vi "Structure Handler.vi"() -> ()   [LabVIEW 2010] (continued)
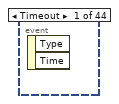
[diagram p4: hidden frame]
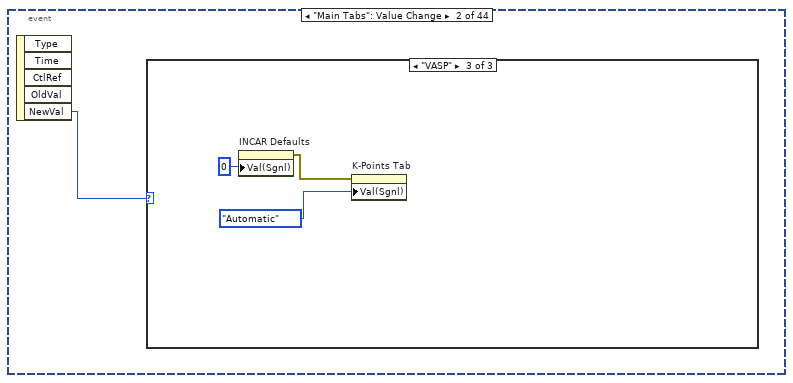
[diagram p5: hidden frame]
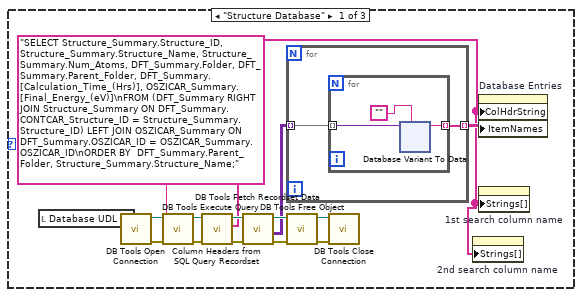
[diagram p6: hidden frame]
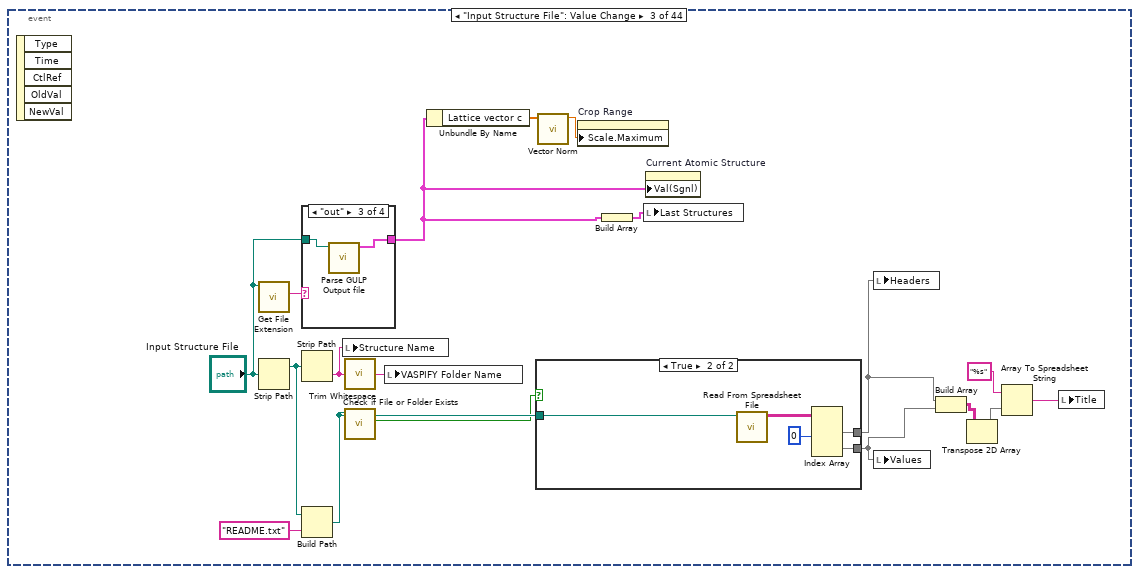
[diagram p8: hidden frame]
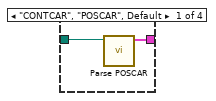
[diagram p10: hidden frame]
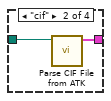
[diagram p11: hidden frame]
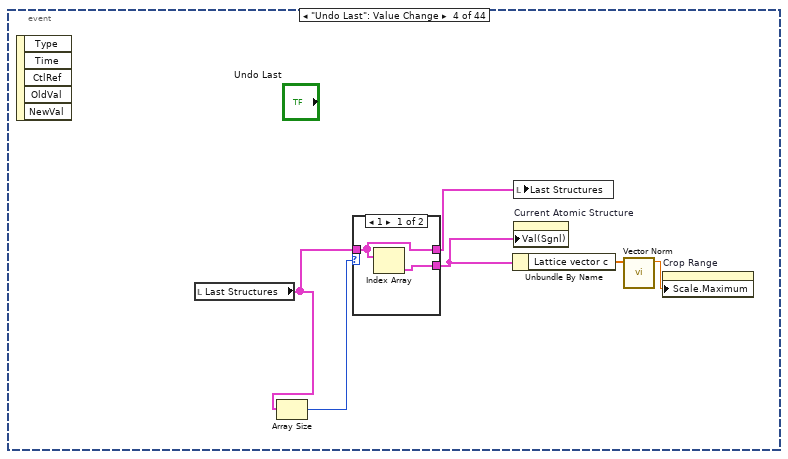
[diagram p13: hidden frame]
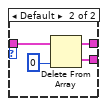
[diagram p14: hidden frame]
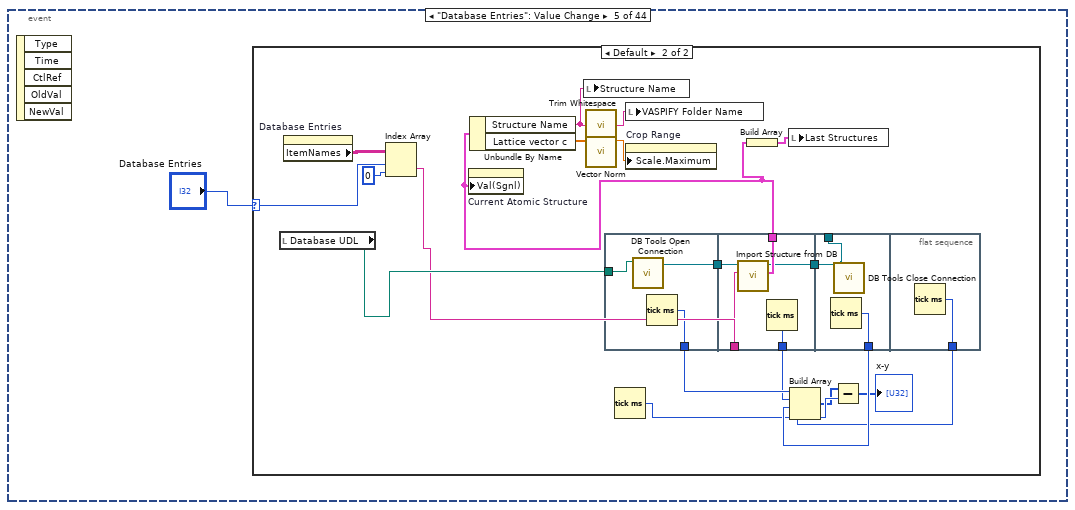
[diagram p15: hidden frame]
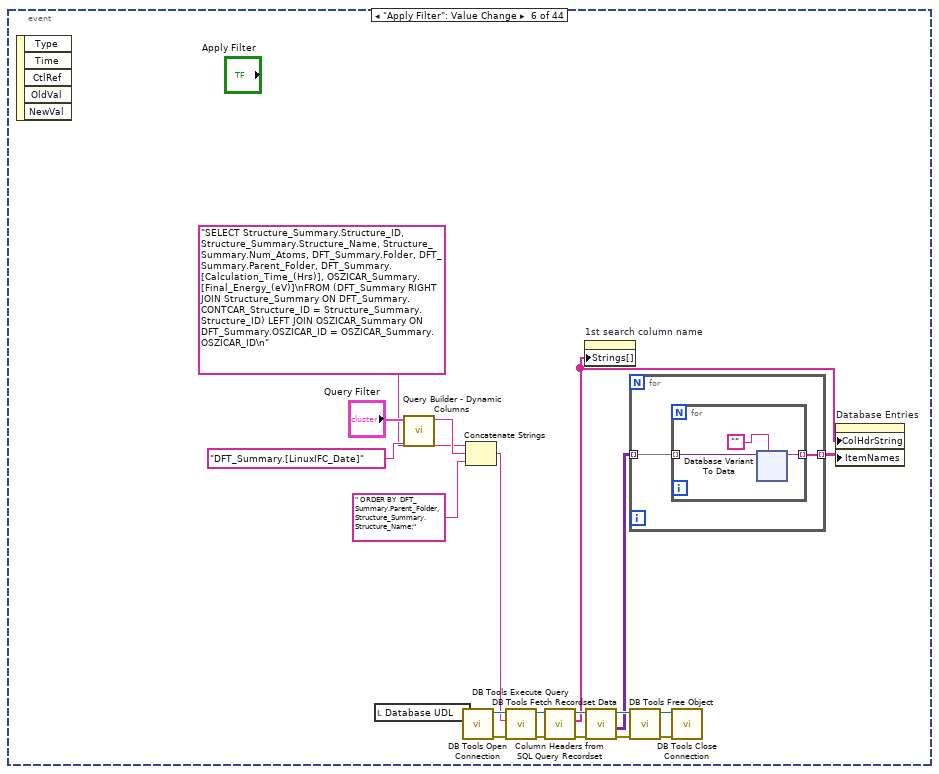
[diagram p17: hidden frame]
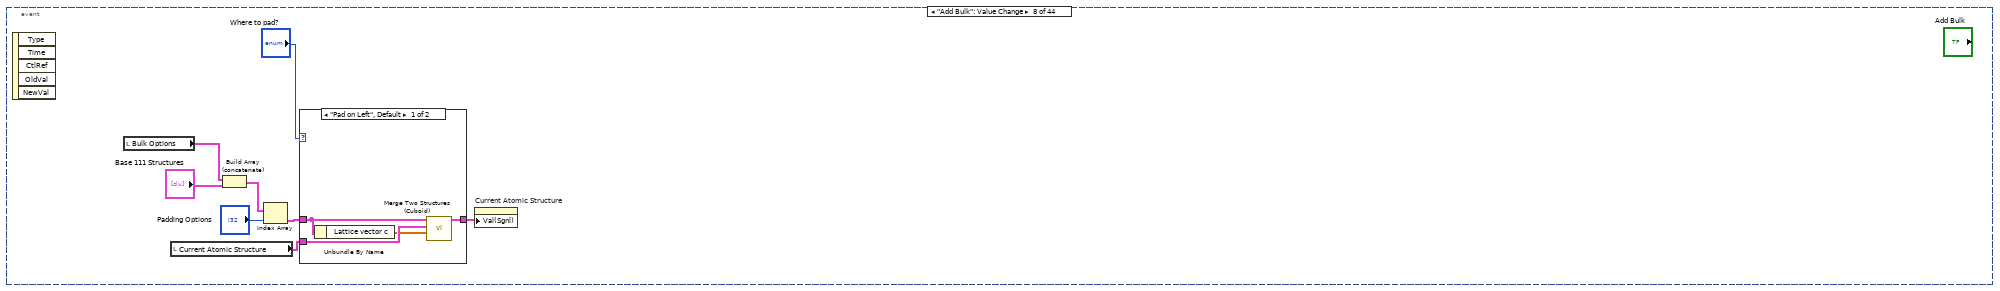
[diagram p19: hidden frame]
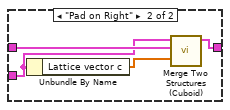
[diagram p20: hidden frame]
                  }
                  frame True {
                    n569 = local read "Atom List"() -> (w1005:i32[])
                    n570 = Search 1D Array(1D array=w1005, element=w1004) -> (index of element=w1003:i32)  [unwired: 1 in]
                    n571 = case shown="Default" w1003 {
                      tunnel: [w1007 w1010] -> w1006
                      tunnel: w1005 -> [w1007 w1009]
                      tunnel: w1004 -> [_ w1008]
                      frame Default {
                      }
                      frame -1 {
                        n572 = Build Array (concatenate)(w1009, w1008) -> (w1010:i32[])
                      }
                    }
                  }
                }
                n573 = property on="Atom List" class="MCListbox (strict)"("Val(Sgnl)"=w986) -> ()  [unwired: 2 in, 2 out]
              }
            }
          }
        }
      }
      event "Make Vacancy": Value Change {
        n574 = event-data() -> ()  [unwired: 1 in, 5 out]
        n575 = local read "Current Atomic Structure"() -> (w1031:T3)
        n576 = Unbundle By Name(w1031) -> ("Atoms Array"=w1032:T20, "# of atoms"=w1028:i32)
        n577 = local read "Atom List"() -> (w1030:i32[])
        n578 = for {
          tunnel: w1032 -> [w1057] mode=indexing
          tunnel: w1030 -> [w1059]
          tunnel: [w1053] -> w1025 mode=indexing
          shift-right: [w1051] -> _
          shift-left: 0 -> [w1052]
          w1058 = dbl[][] []
          n579 = Unbundle By Name(w1057) -> ("Atom Name"=w1056:string, "Positions (Direct)"=w1061:dbl[][], "Positions (Cartesian)"=w1060:dbl[][])
          n580 = for {
            tunnel: w1061 -> [w1069] mode=indexing
            tunnel: w1060 -> [w1066] mode=indexing
            tunnel: w1059 -> [w1071]
            shift-right: [w1065] -> w1054
            shift-left: w1058 -> [w1064]
            shift-right: [w1068] -> w1055
            shift-left: w1058 -> [w1067]
            shift-right: [w1063] -> w1051
            shift-left: w1052 -> [w1062]
            n581 = Search 1D Array(1D array=w1071, element=w1062) -> (index of element=w1070:i32)  [unwired: 1 in]
            n582 = Increment(x=w1062) -> (x+1=w1063:i32)
            n583 = case shown="Default" w1070 {
              tunnel: w1069 -> [_ w1079]
              tunnel: [w1073 w1078] -> w1068
              tunnel: w1067 -> [w1073 w1077]
              tunnel: w1066 -> [_ w1076]
              tunnel: [w1072 w1075] -> w1065
              tunnel: w1064 -> [w1072 w1074]
              frame Default {
              }
              frame -1 {
                n584 = Build Array (concatenate)(w1077, w1079) -> (w1078:dbl[][])
                n585 = Build Array (concatenate)(w1074, w1076) -> (w1075:dbl[][])
              }
            }
          }
          n586 = Bundle(cluster=w1057, "Atom Name"=w1056, "Positions (Direct)"=w1055, "Positions (Cartesian)"=w1054) -> (w1053:T23)
        }
        n587 = Array Size(array=w1030) -> (size(s)=w1029:i32)
        n588 = Subtract(x=w1028, y=w1029) -> (x-y=w1027:i32)
        n589 = Bundle By Name(cluster=w1031, "Atoms Array"=w1025, "# of atoms"=w1027) -> (w1026:T3)
        n590 = local read "Headers"() -> (w1020:string[])
        n591 = local read "Values"() -> (w1021:string[])
        n592 = property on="Current Atomic Structure" class="Clust (strict)"("Val(Sgnl)"=w1026) -> ()  [unwired: 2 in, 2 out]
        n593 = for {
          tunnel: string[] ["Defect Name", "Location"] -> [w1035] mode=indexing
          shift-right: [w1036] -> w1022
          shift-left: w1020 -> [w1037]
          shift-right: [w1033] -> w1023
          shift-left: w1021 -> [w1038]
          tunnel: string[] ["Vacancy", ""] -> [w1034] mode=indexing
          n594 = Search 1D Array(1D array=w1037, element=w1035) -> (index of element=w1039:i32)  [unwired: 1 in]
          n595 = case shown="-1" w1039 {
            selector: w1039 -> [w1043 _]
            tunnel: w1038 -> [w1044 w1047]
            tunnel: [w1042 w1045] -> w1033
            tunnel: w1037 -> [w1041 w1050]
            tunnel: [w1041 w1048] -> w1036
            tunnel: w1035 -> [_ w1049]
            tunnel: w1034 -> [w1040 w1046]
            frame Default {
              n596 = Replace Array Subset(array=w1044, new element=w1040, index=w1043) -> (w1042:string[])
            }
            frame -1 {
              n597 = Build Array (concatenate)(w1047, w1046) -> (w1045:string[])
              n598 = Build Array (concatenate)(w1050, w1049) -> (w1048:string[])
            }
          }
        }
        n599 = local write "Values"(w1023) -> ()
        n600 = local write "Headers"(w1022) -> ()
      }
      event "Replace Atom": Value Change {
        w1088 = dbl[][] []
        n601 = event-data() -> ()  [unwired: 1 in, 5 out]
        n602 = local read "Current Atomic Structure"() -> (w1099:T3)
        n603 = local read "Atom List"() -> (w1098:i32[])
        n604 = Unbundle By Name(w1099) -> ("Atoms Array"=w1100:T20)
        n605 = for {
          tunnel: w1100 -> [w1150] mode=indexing
          tunnel: w1098 -> [w1151]
          tunnel: [w1146] -> w1095 mode=indexing
          shift-right: [w1144] -> _
          shift-left: 0 -> [w1145]
          shift-right: [w1142] -> w1090
          shift-left: w1088 -> [w1140]
          shift-right: [w1141] -> w1089
          shift-left: w1088 -> [w1139]
          w1143 = dbl[][] []
          n606 = Unbundle By Name(w1150) -> ("Atom Name"=w1149:string, "Positions (Direct)"=w1153:dbl[][], "Positions (Cartesian)"=w1152:dbl[][])
          n607 = for {
            tunnel: w1153 -> [w1165] mode=indexing
            tunnel: w1152 -> [w1162] mode=indexing
            tunnel: w1151 -> [w1167]
            shift-right: [w1161] -> w1147
            shift-left: w1143 -> [w1160]
            shift-right: [w1164] -> w1148
            shift-left: w1143 -> [w1163]
            shift-right: [w1159] -> w1144
            shift-left: w1145 -> [w1158]
            shift-right: [w1157] -> w1142
            shift-left: w1140 -> [w1156]
            shift-right: [w1155] -> w1141
            shift-left: w1139 -> [w1154]
            n608 = Search 1D Array(1D array=w1167, element=w1158) -> (index of element=w1166:i32)  [unwired: 1 in]
            n609 = case shown="-1" w1166 {
              tunnel: w1165 -> [w1173 w1183]
              tunnel: [w1175 w1182] -> w1164
              tunnel: w1163 -> [w1175 w1181]
              tunnel: w1162 -> [w1170 w1180]
              tunnel: [w1174 w1179] -> w1161
              tunnel: w1160 -> [w1174 w1178]
              tunnel: [w1172 w1176] -> w1157
              tunnel: w1156 -> [w1171 w1176]
              tunnel: [w1169 w1177] -> w1155
              tunnel: w1154 -> [w1168 w1177]
              frame Default {
                n610 = Build Array (concatenate)(w1171, w1173) -> (w1172:dbl[][])
                n611 = Build Array (concatenate)(w1168, w1170) -> (w1169:dbl[][])
              }
              frame -1 {
                n612 = Build Array (concatenate)(w1181, w1183) -> (w1182:dbl[][])
                n613 = Build Array (concatenate)(w1178, w1180) -> (w1179:dbl[][])
              }
            }
            n614 = Increment(x=w1158) -> (x+1=w1159:i32)
          }
          n615 = Bundle(cluster=w1150, "Atom Name"=w1149, "Positions (Direct)"=w1148, "Positions (Cartesian)"=w1147) -> (w1146:T23)
        }
        n616 = for {
          tunnel: w1095 -> [w1128] mode=indexing
          tunnel: w1090 -> [w1127]
          tunnel: w1089 -> [w1126]
          tunnel: [w1125] -> w1094 mode=indexing
          tunnel: "Replacement Atom" -> [w1124]
          tunnel: [w1123] -> w1087 mode=indexing
          n617 = Unbundle By Name(w1128) -> ("Atom Name"=w1129:string)
          n618 = Equal?(x=w1124, y=w1129) -> (x = y?=w1123:bool)
          n619 = case shown="True" w1123 {
            tunnel: w1128 -> [w1130 w1134]
            tunnel: w1127 -> [_ w1137]
            tunnel: w1126 -> [_ w1135]
            tunnel: [w1130 w1131] -> w1125
            frame False {
            }
            frame True {
              n620 = Unbundle By Name(w1134) -> ("Positions (Direct)"=w1138:dbl[][], "Positions (Cartesian)"=w1136:dbl[][])
              n621 = Build Array (concatenate)(w1138, w1137) -> (w1132:dbl[][])
              n622 = Build Array (concatenate)(w1136, w1135) -> (w1133:dbl[][])
              n623 = Bundle By Name(cluster=w1134, "Positions (Direct)"=w1132, "Positions (Cartesian)"=w1133) -> (w1131:T23)
            }
          }
        }
        n624 = Bundle("Replacement Atom"="Replacement Atom", w1090, w1089) -> (w1091:T29)  [unwired: 1 in]
        n625 = Or Array Elements(Boolean array=w1087) -> (logical OR=w1086:bool)
        n626 = case shown="False" w1086 {
          tunnel: w1094 -> [w1121 w1122]
          tunnel: [w1120 w1122] -> w1093
          tunnel: w1091 -> [w1119 _]
          frame False {
            n627 = Build Array (concatenate)(w1121, w1119) -> (w1120:T30)
          }
          frame True {
          }
        }
        n628 = Bundle By Name(cluster=w1099, "Atoms Array"=w1093) -> (w1097:T3)
        n629 = property on="Current Atomic Structure" class="Clust (strict)"("Val(Sgnl)"=w1097) -> ()  [unwired: 2 in, 2 out]
        n630 = local read "Headers"() -> (w1082:string[])
        n631 = local read "Values"() -> (w1083:string[])
        n632 = for {
          tunnel: string[] ["Defect Name", "Location"] -> [w1103] mode=indexing
          shift-right: [w1104] -> w1084
          shift-left: w1082 -> [w1105]
          shift-right: [w1101] -> w1085
          shift-left: w1083 -> [w1106]
          tunnel: string[] ["Substitutional", ""] -> [w1102] mode=indexing
          n633 = Search 1D Array(1D array=w1105, element=w1103) -> (index of element=w1107:i32)  [unwired: 1 in]
          n634 = case shown="-1" w1107 {
            selector: w1107 -> [w1111 _]
            tunnel: w1106 -> [w1112 w1115]
            tunnel: [w1110 w1113] -> w1101
            tunnel: w1105 -> [w1109 w1118]
            tunnel: [w1109 w1116] -> w1104
            tunnel: w1103 -> [_ w1117]
            tunnel: w1102 -> [w1108 w1114]
            frame Default {
              n635 = Replace Array Subset(array=w1112, new element=w1108, index=w1111) -> (w1110:string[])
            }
            frame -1 {
              n636 = Build Array (concatenate)(w1115, w1114) -> (w1113:string[])
              n637 = Build Array (concatenate)(w1118, w1117) -> (w1116:string[])
            }
          }
        }
        n638 = local write "Values"(w1085) -> ()
        n639 = local write "Headers"(w1084) -> ()
      }
      event "Add Interstitial": Value Change {
        w1202 = dbl[] [0.0, 0.0, 0.0]
        n640 = event-data() -> ()  [unwired: 1 in, 5 out]
        n641 = local read "Current Atomic Structure"() -> (w1194:T3)
        n642 = local read "Headers"() -> (w1189:string[])
        n643 = local read "Values"() -> (w1188:string[])
        n644 = Unbundle By Name(w1194) -> ("Atoms Array"=w1203:T20, "# of atoms"=w1192:i32)
        n645 = for {
          tunnel: string[] ["Defect Name", "Location"] -> [w1207] mode=indexing
          shift-right: [w1208] -> w1187
          shift-left: w1189 -> [w1209]
          shift-right: [w1205] -> w1186
          shift-left: w1188 -> [w1210]
          tunnel: string[] ["Interstitial", ""] -> [w1206] mode=indexing
          n646 = Search 1D Array(1D array=w1209, element=w1207) -> (index of element=w1211:i32)  [unwired: 1 in]
          n647 = case shown="-1" w1211 {
            selector: w1211 -> [w1215 _]
            tunnel: w1210 -> [w1216 w1219]
            tunnel: [w1214 w1217] -> w1205
            tunnel: w1209 -> [w1213 w1222]
            tunnel: [w1213 w1220] -> w1208
            tunnel: w1207 -> [_ w1221]
            tunnel: w1206 -> [w1212 w1218]
            frame Default {
              n648 = Replace Array Subset(array=w1216, new element=w1212, index=w1215) -> (w1214:string[])
            }
            frame -1 {
              n649 = Build Array (concatenate)(w1219, w1218) -> (w1217:string[])
              n650 = Build Array (concatenate)(w1222, w1221) -> (w1220:string[])
            }
          }
        }
        n651 = local read "Atom List"() -> (w1190:i32[])
        n652 = for {
          tunnel: w1203 -> [w1229] mode=indexing
          tunnel: w1190 -> [w1230]
          shift-right: [w1223] -> _
          shift-left: 0 -> [w1228]
          shift-right: [w1227] -> w1200
          shift-left: w1202 -> [w1225]
          shift-right: [w1226] -> w1199
          shift-left: w1202 -> [w1224]
          tunnel: [w1223] -> _ mode=indexing
          n653 = Unbundle By Name(w1229) -> ("Positions (Direct)"=w1232:dbl[][], "Positions (Cartesian)"=w1231:dbl[][])  [unwired: 1 out]
          n654 = for {
            tunnel: w1232 -> [w1240] mode=indexing
            tunnel: w1231 -> [w1239] mode=indexing
            tunnel: w1230 -> [w1242]
            shift-right: [w1233] -> w1223
            shift-left: w1228 -> [w1238]
            shift-right: [w1237] -> w1227
            shift-left: w1225 -> [w1236]
            shift-right: [w1235] -> w1226
            shift-left: w1224 -> [w1234]
            n655 = Search 1D Array(1D array=w1242, element=w1238) -> (index of element=w1241:i32)  [unwired: 1 in]
            n656 = case shown="Default" w1241 {
              tunnel: w1240 -> [w1247 _]
              tunnel: w1239 -> [w1244 _]
              tunnel: [w1246 w1249] -> w1237
              tunnel: w1236 -> [w1248 w1249]
              tunnel: [w1243 w1250] -> w1235
              tunnel: w1234 -> [w1245 w1250]
              frame Default {
                n657 = Add(x=w1248, y=w1247) -> (x+y=w1246:dbl[])
                n658 = Add(x=w1245, y=w1244) -> (x+y=w1243:dbl[])
              }
              frame -1 {
              }
            }
            n659 = Increment(x=w1238) -> (x+1=w1233:i32)
          }
        }
        n660 = Array Size(array=w1190) -> (size(s)=w1198:i32)
        n661 = Increment(x=w1192) -> (x+1=w1191:i32)
        n662 = local write "Headers"(w1187) -> ()
        n663 = local write "Values"(w1186) -> ()
        n664 = local read "Replacement Atom"() -> (w1204:string)
        n665 = Divide(x=w1200, y=w1198) -> (x/y=w1197:dbl[])
        n666 = Divide(x=w1199, y=w1198) -> (x/y=w1196:dbl[])
        n667 = for {
          tunnel: w1203 -> [w1256] mode=indexing
          tunnel: w1197 -> [w1255]
          tunnel: w1196 -> [w1254]
          tunnel: [w1253] -> w1195 mode=indexing
          tunnel: w1204 -> [w1252]
          n668 = Unbundle By Name(w1256) -> ("Atom Name"=w1257:string)
          n669 = Equal?(x=w1252, y=w1257) -> (x = y?=w1251:bool)
          n670 = case shown="True" w1251 {
            tunnel: w1256 -> [w1258 w1262]
            tunnel: w1255 -> [_ w1265]
            tunnel: w1254 -> [_ w1263]
            tunnel: [w1258 w1259] -> w1253
            frame False {
            }
            frame True {
              n671 = Unbundle By Name(w1262) -> ("Positions (Direct)"=w1266:dbl[][], "Positions (Cartesian)"=w1264:dbl[][])
              n672 = Build Array (concatenate)(w1266, w1265) -> (w1260:dbl[][])
              n673 = Build Array (concatenate)(w1264, w1263) -> (w1261:dbl[][])
              n674 = Bundle By Name(cluster=w1262, "Positions (Direct)"=w1260, "Positions (Cartesian)"=w1261) -> (w1259:T23)
            }
          }
        }
        n675 = Bundle By Name(cluster=w1194, "Atoms Array"=w1195, "# of atoms"=w1191) -> (w1193:T3)
        n676 = property on="Current Atomic Structure" class="Clust (strict)"("Val(Sgnl)"=w1193) -> ()  [unwired: 2 in, 2 out]
      }
      event "Make defect pair": Value Change {
        n677 = event-data() -> ()  [unwired: 1 in, 5 out]
        n678 = local read "Current Atomic Structure"() -> (w1269:T3)
        n679 = call "Make Defect Pair.vi"("Maximum Distnce"="Maximum Distnce", "Minimum Distance"="Minimum Distance", "Defect 2"="Defect 2", "Defect 1"="Defect 1", "Defect 1 Atom Index"="Defect 1 Atom Index", "Input Structure"=w1269) -> ("Defectuous Structure"=w1270:T3)  [unwired: 2 in, 3 out]
        n680 = property on="Current Atomic Structure" class="Clust (strict)"("Val(Sgnl)"=w1270) -> ()  [unwired: 2 in, 2 out]
      }
      event "Max Bond Length", "Axis": Value Change {
        n681 = event-data() -> ()  [unwired: 1 in, 5 out]
        n682 = local read "Current Atomic Structure"() -> (w1278:T3)
        n683 = call "Find all Bonds in Structure.vi"("Max Bond Length"="Max Bond Length", "Structure"=w1278) -> ("Bonds"=w1277:T31)  [unwired: 9 in]
        n684 = for {
          tunnel: w1277 -> [w1285] mode=indexing
          tunnel: "Axis" -> [w1283]
          tunnel: [w1280] -> w1275 mode=indexing
          n685 = Unbundle By Name(w1285) -> ("Bond Center Position"=w1284:dbl[], "Bond Length (A)"=w1281:dbl)
          n686 = Index Array(array=w1284, index=w1283) -> (element=w1282:dbl)
          n687 = Bundle("Numeric"=w1282, "Bond Length (A)"=w1281) -> (w1280:cluster{"Numeric":dbl, "Bond Length (A)":dbl})  [unwired: 1 in]
        }
        n688 = Sort 1D Array(array=w1275) -> (sorted array=→"System XY Graph":cluster{"Numeric":dbl, "Bond Length (A)":dbl}[])
      }
      event "Map to [0,1)": Value Change {
        n689 = event-data() -> ()  [unwired: 1 in, 5 out]
        n690 = local read "Current Atomic Structure"() -> (w1287:T3)
        n691 = call "Map Structure to [0,1).vi"("Structure"=w1287) -> ("Structure mapped to [0,1)"=w1286:T32)  [unwired: 10 in]
        n692 = property on="Current Atomic Structure" class="Clust (strict)"("Val(Sgnl)"=w1286) -> ()  [unwired: 2 in, 2 out]
      }
      event "Remove Close Atoms": Value Change {
        n693 = event-data() -> ()  [unwired: 1 in, 5 out]
        n694 = local read "Current Atomic Structure"() -> (w1291:T3)
        n695 = call "Remove Close Atoms.vi"("Minimally Allowable Distance (A)"="Minimally Allowable Distance (A)", "Structure"=w1291) -> ("# of Atoms Removed"=→"# of Atoms Removed":i32, "Structure with atoms removed"=w1290:T3)  [unwired: 8 in]
        n696 = property on="Current Atomic Structure" class="Clust (strict)"("Val(Sgnl)"=w1290) -> ()  [unwired: 2 in, 2 out]
      }
      event "Load in VESTA": Value Change {
        n697 = event-data() -> ()  [unwired: 1 in, 5 out]
        n698 = local read "Current Atomic Structure"() -> (w1292:T3)
        n699 = call "Load Structure in VESTA.vi"("Atomic Structure"=w1292) -> ()  [unwired: 11 in]
      }
    }
  }
  n700 = call <vilib>:"Create Object.vi"("Name"="Base") -> ("error out"=w1:errorcluster, "Scene:New Object"=w2:refnum<vi>)  [unwired: 1 in, 8 out]
  n701 = local write "Base Object"(w2) -> ()
  n702 = disable-structure shown="Disabled" {
    disable-tunnel: w1 -> [w1294 _]
    frame Disabled {
      n703 = property on="Current Atomic Structure" class="Clust (strict)"(error in=w1294, "Val(Sgnl)"=T3 {"Structure Name"="(60.0) twist [1,1,1] [1,1,1+0.0tilt] (0.00,0.00,0.00)T GB", "Lattice vector a"=[4.678066827442777, 0.0, 0.0], "Lattice vector b"=[0.0, 8.10264942633344, 0.0], "Lattice vector c"=[0.0, 0.0, 23.0], "Atoms Array"=[{"Atom Name"="Cd", "Positions (Direct)"=[[0.0, 5.4807901278164903e-17, -0.000893984567927683], [0.0, 0.0, 0.4991060154320723], [0.0, 0.3333333333333333, 0.3321413539094297], [0.0, 0.6666666666666666, 0.16607067695471486], [0.4999999999999999, 0.16666666666666666, 0.16607067695471486], [0.5, 0.5, -0.000893984567927683], [0.5, 0.5, 0.4991060154320723], [0.4999999999999999, 0.8333333333333331, 0.3321413539094297], [0.9999999999999998, 0.3333333333333333, 0.3321413539094297], [0.9999999999999998, 0.6666666666666667, 0.16607067695471486], [0.0, 0.33333333333333326, 0.6660706769547148], [0.0, 0.6666666666666666, 0.8321413539094297], [0.5, 0.16666666666666674, 0.8321413539094297], [0.5, 0.8333333333333333, 0.6660706769547148]], "Positions (Cartesian)"=[[0.0, 4.440892098500626e-16, -0.02056164506233671], [0.0, 0.0, 11.479438354937663], [0.0, 2.700883142111146, 7.639251139916884], [0.0, 5.401766284222292, 3.819625569958442], [2.339033413721388, 1.350441571055573, 3.819625569958442], [2.3390334137213884, 4.05132471316672, -0.02056164506233671], [2.3390334137213884, 4.05132471316672, 11.479438354937663], [2.339033413721388, 6.752207855277865, 7.639251139916884], [4.678066827442776, 2.700883142111146, 7.639251139916884], [4.678066827442776, 5.401766284222293, 3.819625569958442], [0.0, 2.7008831421111457, 15.319625569958442], [0.0, 5.401766284222292, 19.139251139916883], [2.3390334137213884, 1.3504415710555737, 19.139251139916883], [2.3390334137213884, 6.752207855277866, 15.319625569958442]]}, {"Atom Name"="Te", "Positions (Direct)"=[[0.0, 0.0, 0.12455300771603617], [0.0, 0.33333333333333337, 0.45669436162546595], [0.0, 0.6666666666666666, 0.29062368467075106], [0.4999999999999999, 0.16666666666666663, 0.29062368467075106], [0.4999999999999999, 0.4999999999999999, 0.12455300771603621], [0.4999999999999999, 0.8333333333333331, 0.45669436162546595], [0.9999999999999998, 5.4807901278164903e-17, 0.12455300771603621], [0.9999999999999998, 0.3333333333333333, 0.45669436162546595], [0.9999999999999998, 0.6666666666666669, 0.29062368467075106], [0.0, 1.1331166295920983e-17, 0.6245530077160362], [0.0, 0.3333333333333333, 0.7906236846707511], [0.0, 0.6666666666666666, 0.9566943616254658], [0.0, 0.9999999999999998, 0.6245530077160362], [0.4999999999999999, 0.1666666666666668, 0.9566943616254658], [0.4999999999999999, 0.8333333333333334, 0.7906236846707511], [0.5000000000000001, 0.5, 0.6245530077160362]], "Positions (Cartesian)"=[[0.0, 0.0, 2.864719177468832], [0.0, 2.7008831421111466, 10.503970317385717], [0.0, 5.401766284222292, 6.684344747427274], [2.339033413721388, 1.3504415710555728, 6.684344747427275], [2.339033413721388, 4.051324713166719, 2.864719177468833], [2.339033413721388, 6.752207855277865, 10.503970317385717], [4.678066827442776, 4.440892098500626e-16, 2.864719177468833], [4.678066827442776, 2.700883142111146, 10.503970317385717], [4.678066827442776, 5.401766284222294, 6.684344747427275], [0.0, 9.181246808733296e-17, 14.364719177468832], [0.0, 2.700883142111146, 18.184344747427275], [0.0, 5.401766284222292, 22.003970317385715], [0.0, 8.102649426333437, 14.364719177468833], [2.339033413721388, 1.3504415710555742, 22.003970317385715], [2.339033413721388, 6.752207855277867, 18.184344747427275], [2.339033413721389, 4.05132471316672, 14.364719177468833]]}], "# of atoms"=30} ("Grain Boundary")) -> ()  [unwired: 1 in, 2 out]
    }
    frame Enabled {
    }
  }
